vi "joystick arc to vector.vi"(0 "Jx":dbl(slide) scale=-1.0..1.0, 2 "Jy":dbl(slide) scale=-1.0..1.0, 9 "sector width (deg)":dbl(ring)=45.0 format="%#_13g" items=["4-sectors"=90.0, "6-sectors"=60.0, "8-sectors"=45.0]) -> (14 "Jx":dbl, 16 "Jy":dbl, 17 "theta (deg)":dbl, 19 "theta (rad)":dbl)   [LabVIEW 2023]
uses:
  <vilib>/Analysis/coordinate.llb/Angle Units.ctl
  <vilib>/Analysis/coordinate.llb/Angle Range (Degree).ctl
  <vilib>/Analysis/coordinate.llb/Wrap Angle (scalar).vi
  <vilib>/Analysis/coordinate.llb/Check for Included Angle (scalar).vi
  <vilib>/Analysis/coordinate.llb/Absolute Angle Difference (scalar).vi
  <vilib>/Analysis/coordinate.llb/Set Angle Unit.vi
  <vilib>/Analysis/NI_AAL_Angle.lvlib
panel:
  out "arc center":dbl[](array[numeric])
  out "Array":bool[](array[boolean])
  out "angle (deg)":dbl
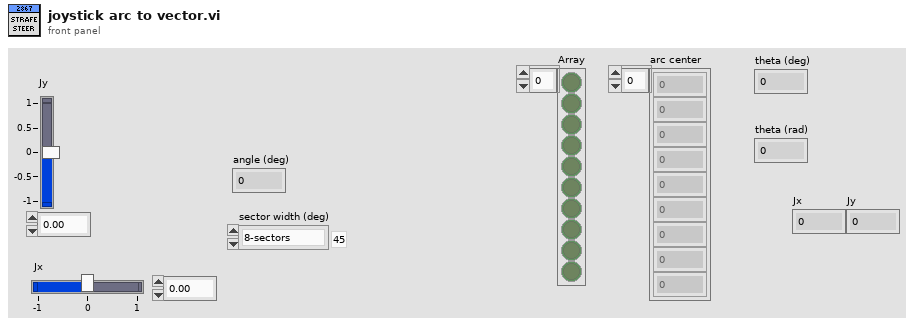
[diagram p1: front panel]
types:
  T1 = typedef "NI_AAL_Angle.lvlib/Angle Range (Degree).ctl" = u16
  T2 = typedef "NI_AAL_Angle.lvlib/Angle Units.ctl" = i32
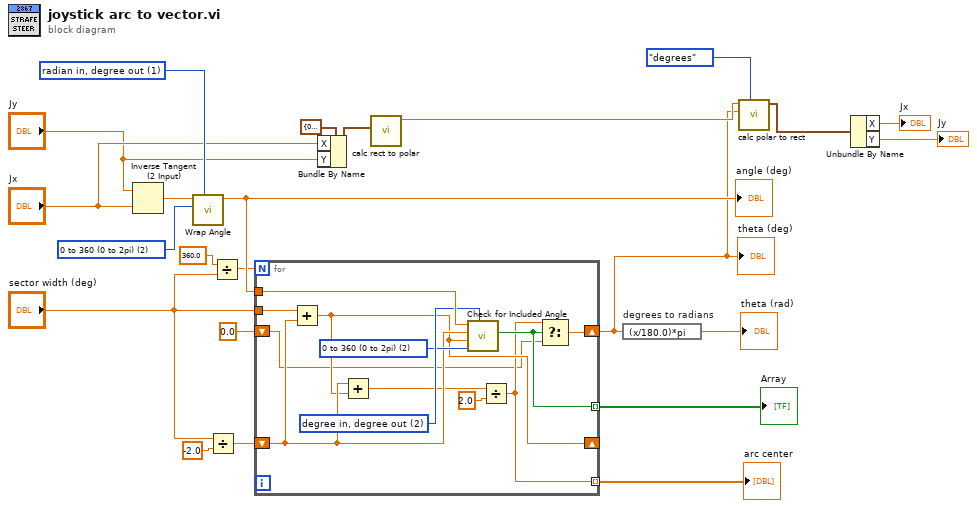
[diagram p0: block diagram]
diagram:
  w21 = T1 2 items=["none", "-180 to 180 (-pi to pi)", "0 to 360 (0 to 2pi)"] ("angle range")
  w22 = T2 1 items=["radian in, radian out", "radian in, degree out", "degree in, degree out", "degree in, radian out"] ("angle units")
  n1 = Inverse Tangent (2 Input)(1:"Jx", 2:"Jy") -> (0:w23:dbl)
  n2 = call-poly <vilib>:"Wrap Angle.vi"("angle units"=w22, "angle range"=w21, "angle in"=w23) -> ("angle out"=w20:dbl)  [unwired: 7 in, 1 out]
  "angle (deg)" <- w20
  n3 = Divide(x="sector width (deg)", y=-2.0) -> (x/y=w16:dbl)
  n4 = Divide(x=360.0, y="sector width (deg)") -> (x/y=w18:dbl)
  n5 = for {
    N: w18 -> [_]
    shift-right: [w30] -> _
    shift-left: w16 -> [w31]
    tunnel: w20 -> [w35]
    tunnel: "sector width (deg)" -> [w32]
    tunnel: [w26] -> w17 mode=indexing
    tunnel: [w25] -> w13 mode=indexing
    shift-right: [w27] -> w4
    shift-left: 0.0 -> [w24]
    w33 = T1 2 items=["none", "-180 to 180 (-pi to pi)", "0 to 360 (0 to 2pi)"] ("output angle range")
    w34 = T2 2 items=["radian in, radian out", "radian in, degree out", "degree in, degree out", "degree in, radian out"] ("angle units")
    n6 = Add(x=w32, y=w31) -> (x+y=w30:dbl)
    n7 = Add(x=w31, y=w30) -> (x+y=w29:dbl)
    n8 = call-poly <vilib>:"Check for Included Angle.vi"("angle units"=w34, "output angle range"=w33, "end angle"=w30, "start angle"=w31, "angle in"=w35) -> ("in range?"=w26:bool)  [unwired: 4 in, 2 out]
    n9 = Divide(x=w29, y=2.0) -> (x/y=w25:dbl)
    n10 = Select(t=w25, s=w26, f=w24) -> (s? t:f=w27:dbl)
  }
  "Array" <- w17
  "arc center" <- w13
  "theta (deg)" <- w4
  n11 = Bundle By Name(cluster=cluster{"X":dbl, "Y":dbl} {"X"=0.0, "Y"=0.0} ("XY"), "X"="Jx", "Y"="Jy") -> (w9:cluster{"X":dbl, "Y":dbl})
  n12 = call "calc rect to polar.vi"("XY"=w9) -> ("Magnitude"=w5:dbl)  [unwired: 8 in, 2 out]
  n13 = expression code="(x/180.0)*pi" "degrees to radians"(w4) -> (→"theta (rad)":dbl)
  n14 = call "calc polar to rect.vi"("units"=enum16{"degrees", "radians"}."degrees", "angle"=w4, "mag"=w5) -> ("XY"=w3:cluster{"X":dbl, "Y":dbl})  [unwired: 8 in]
  n15 = Unbundle By Name(w3) -> ("X"=→"Jx":dbl, "Y"=→"Jy":dbl)
